vi "Async Read Volt.vi"(8 "error in (no error)":errorcluster, 11 "Async Data out":T1={"Hardware"={"Switch Device"="", "DMM Device"="", "DMM -> Switch Trigger"=0, "Switch -> DMM Trigger"=0, "Sample Interval (sec)"=0.0, "Current Samples"=0, "Current Limit"=1.2, "Current Resolution"=5.5, "Auto-Read"=FALSE, "Keep Values"=FALSE}, "Communication"={"Status Q"=refnum, "Command Q"=refnum, "Voltage FIFO"=refnum, "Voltage Buffer"=[], "Current FIFO"=refnum, "Current Buffer"=[], "Async Events"=refnum}} {"Hardware"."Current Resolution" items=["3 1/2"=3.5, "4 1/2"=4.5, "5 1/2"=5.5, "6 1/2"=6.5, "7 1/2"=7.5]; "Hardware"."Sample Interval (sec)" format="%.2f"}) -> (0 "error out":errorcluster)   [LabVIEW 2011, in "Switch-DMM Custom Device.lvlib"]
uses:
  Switch-DMM Custom Device.lvlib
  Controls/Async Data.ctl
  Controls/Hardware.ctl
  <instrlib>/niDMM/nidmm.llb/niDMM Resolution in Digits.ctl
  Controls/Communication.ctl
  Controls/Async Status.ctl
  Controls/Async State.ctl
  Controls/Async Command.ctl
  Controls/Async Events.ctl
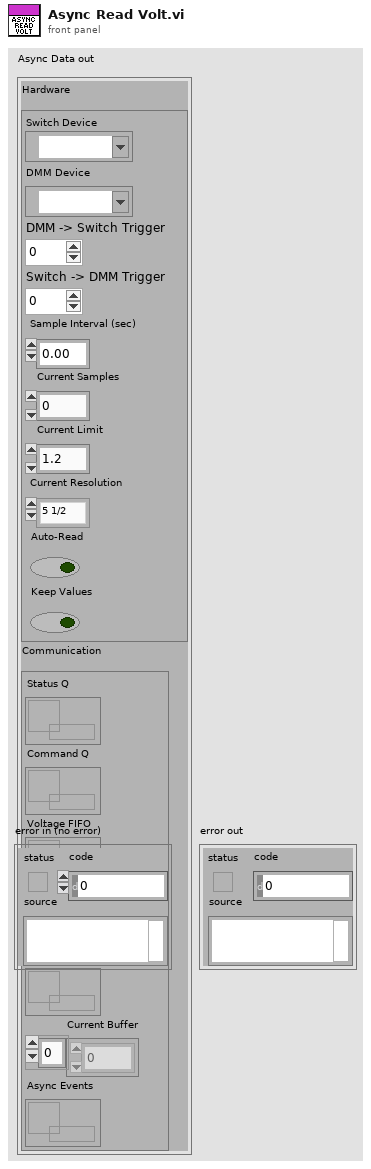
[diagram p1: front panel]
types:
  T1 = typedef "Switch-DMM Custom Device.lvlib/Async Data.ctl" = cluster{"Hardware":T2, "Communication":T4}
  T2 = typedef "Switch-DMM Custom Device.lvlib/Hardware.ctl" = cluster{"Switch Device":refnum<k15>, "DMM Device":refnum<k15>, "DMM -> Switch Trigger":u16, "Switch -> DMM Trigger":u16, "Sample Interval (sec)":dbl, "Current Samples":i32, "Current Limit":dbl, "Current Resolution":T3, "Auto-Read":bool, "Keep Values":bool}
  T3 = typedef "niDMM Resolution in Digits.ctl" = dbl
  T4 = typedef "Switch-DMM Custom Device.lvlib/Communication.ctl" = cluster{"Status Q":refnum<queue>, "Command Q":refnum<queue>, "Voltage FIFO":refnum<k33>, "Voltage Buffer":dbl[], "Current FIFO":refnum<k33>, "Current Buffer":dbl[], "Async Events":refnum<queue>}
  T5 = typedef "Switch-DMM Custom Device.lvlib/Async Events.ctl" = enum16{"None", "Over Current", "Volt Read Done"}
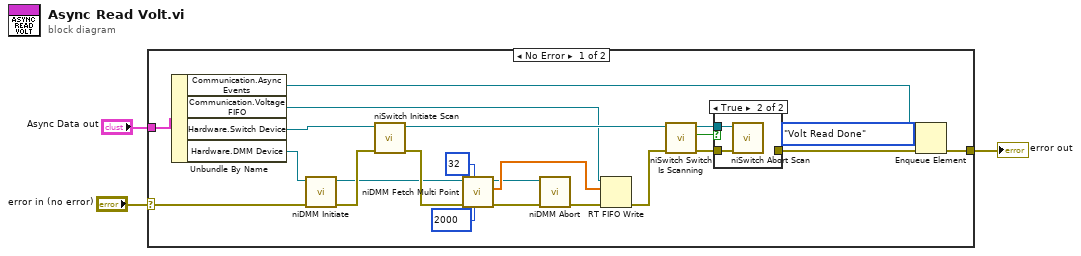
[diagram p0: block diagram]
diagram:
  n1 = case shown="No Error" "error in (no error)" {
    selector: "error in (no error)" -> [w9 w30]
    tunnel: [w6 w30] -> w3
    tunnel: "Async Data out" -> [w20 _]
    frame No Error {
      n2 = Unbundle By Name(w20) -> ("Communication.Async Events"=w5:refnum<queue>, "Communication.Voltage FIFO"=w8:refnum<k33>, "Hardware.Switch Device"=w21:refnum<k15>, "Hardware.DMM Device"=w22:refnum<k15>)
      n3 = call <instrlib>:"niDMM Initiate.vi"("error in (no error)"=w9, "instrument handle"=w22) -> ("error out"=w18:errorcluster, "instrument handle out"=w17:refnum<k15>)  [unwired: 8 out]
      n4 = call <instrlib>:"niSwitch Initiate Scan.vi"("error in (no error)"=w18, "instrument handle"=w21) -> ("error out"=w19:errorcluster, "instrument handle out"=w10:refnum<k15>)  [unwired: 8 out]
      n5 = call <instrlib>:"niDMM Fetch Multi Point.vi"("Maximum Time (msec)"=2000, "Number to Fetch"=32, "error in (no error)"=w19, "instrument handle"=w17) -> ("error out"=w24:errorcluster, "Measurements"=w23:dbl[], "instrument handle out"=w14:refnum<k15>)  [unwired: 5 out]
      n6 = call <instrlib>:"niDMM Abort.vi"("error in (no error)"=w24, "instrument handle"=w14) -> ("error out"=w25:errorcluster)  [unwired: 9 out]
      n7 = RT FIFO Write(0:w8, 1:w23, 3:w25) -> (11:w26:errorcluster)  [unwired: 2 in, 3 out]
      n8 = call <instrlib>:"niSwitch Switch Is Scanning.vi"("error in (no error)"=w26, "instrument handle"=w10) -> ("error out"=w12:errorcluster, "is scanning"=w13:bool, "instrument handle out"=w11:refnum<k15>)  [unwired: 7 in]
      n9 = case shown="True" w13 {
        tunnel: w12 -> [w27 w29]
        tunnel: w11 -> [_ w28]
        tunnel: [w27 _] -> w7
        frame False {
        }
        frame True {
          n10 = call <instrlib>:"niSwitch Abort Scan.vi"("error in (no error)"=w29, "instrument handle"=w28) -> ()  [unwired: 10 out]
        }
      }
      n11 = Enqueue Element(queue=w5, element=Async_Events."Volt Read Done", error in (no error)=w7) -> (error out=w6:errorcluster)  [unwired: 1 in, 2 out]
    }
    frame Error {
    }
  }
  "error out" <- w3
